vi "MotionMagicGoTo.vi"(7 "Reset":bool, 8 "error in (no error)":errorcluster, 9 "Offset(deg)":dbl, 10 "Distance(in)":dbl, 11 "Pod Drive in":refnum<class "Pod Drive.lvclass">) -> (0 "error out":errorcluster, 2 "Enum":T1=enum."ArcToTarget", 3 "Pod Drive out":refnum<class "Pod Drive.lvclass">)   [LabVIEW 2018, in "Drive.lvlib" / "Pod Drive.lvclass"]
uses:
  Pod Drive.lvclass
  Controls/AutoDeliverStateMachine.ctl
  <vilib>/Rock Robotics/WPI/ThirdParty/Phoenix-LabVIEW/Motor Controller/Controls/CTRE_Phoenix_MotorControl_ControlMode.ctl
  Pod Drive.lvclass/Pod Drive.ctl
  <vilib>/Rock Robotics/WPI/ThirdParty/Phoenix-LabVIEW/Motor Controller/Get/CTRE_Phoenix_MotorController_GetSelectedSensorData.vi
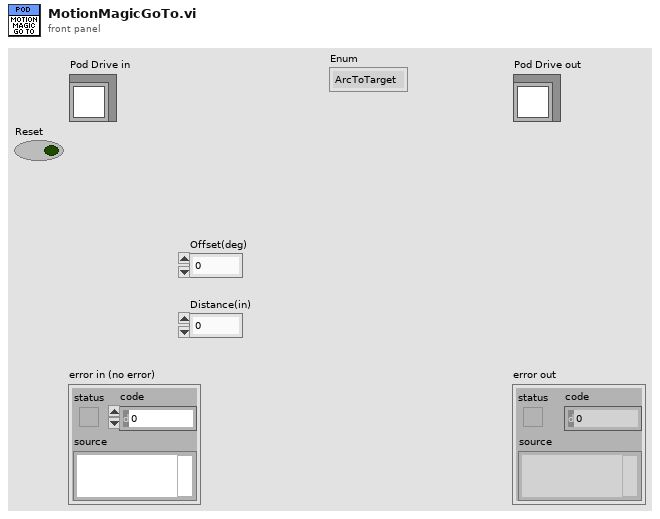
[diagram p1: front panel]
types:
  T1 = typedef "AutoDeliverStateMachine.ctl" = enum16{"Finish", "ArcToTarget", "TurnToTarget"}
  T2 = enum16{"DemandType_Neutral", "DemandType_AuxPID", "DemandType_ArbitraryFeedForward"}
  T3 = typedef "CTRE_Phoenix_MotorControl_ControlMode.ctl" = u16
  T4 = typedef "WPI_MotorControlDeviceRef.ctl" = cluster{"DeviceStatus":errorcluster, "Type":T5, "PWM":cluster{"PWM Channel":T6, "DeadBand":T7}, "CAN":cluster{"Device Number":u8, "SetOutput VI Ref":variant, "GetOutput VI Ref":variant, "Enable VI Ref":variant, "Disable VI Ref":variant, "Data":variant}, "Invert":bool, "DIO PWM":cluster{"PWM \"Enable\" Channel":T6, "DIOChannel":T8, "PWM Rate":dbl}}
  T5 = typedef "WPI_MotorControlType.ctl" = enum16{"PWM", "CAN", "DIO PWM"}
  T6 = typedef "FPGA_DIOPWMChannel.ctl" = enum8{"PWM 0", "PWM 1", "PWM 2", "PWM 3", "PWM 4", "PWM 5", "PWM 6", "PWM 7", "PWM 8", "PWM 9", "PWM MXP 0", "PWM MXP 1", "PWM MXP 2", "PWM MXP 3", "PWM MXP 4", "PWM MXP 5", "PWM MXP 6", "PWM MXP 7", "PWM MXP 8", "PWM MXP 9", "Invalid"}
  T7 = typedef "WPI_PWMDeadband.ctl" = cluster{"Name":string, "maxPositivePwm":i32, "minPositivePwm":i32, "centerPwm":i32, "maxNegativePwm":i32, "minNegativePwm":i32, "angularRange":u16}
  T8 = typedef "FPGA_DIOChannel.ctl" = enum8{"DIO 0", "DIO 1", "DIO 2", "DIO 3", "DIO 4", "DIO 5", "DIO 6", "DIO 7", "DIO 8", "DIO 9", "DIO MXP 0", "DIO MXP 1", "DIO MXP 2", "DIO MXP 3", "DIO MXP 4", "DIO MXP 5", "DIO MXP 6", "DIO MXP 7", "DIO MXP 8", "DIO MXP 9", "DIO MXP 10", "DIO MXP 11", "DIO MXP 12", "DIO MXP 13", "DIO MXP 14", "DIO MXP 15", "SPI Port CS1", "SPI Port CS2", "SPI Port CS3", "SPI Port MISO", "SPI Port MOSI", "Invalid"}
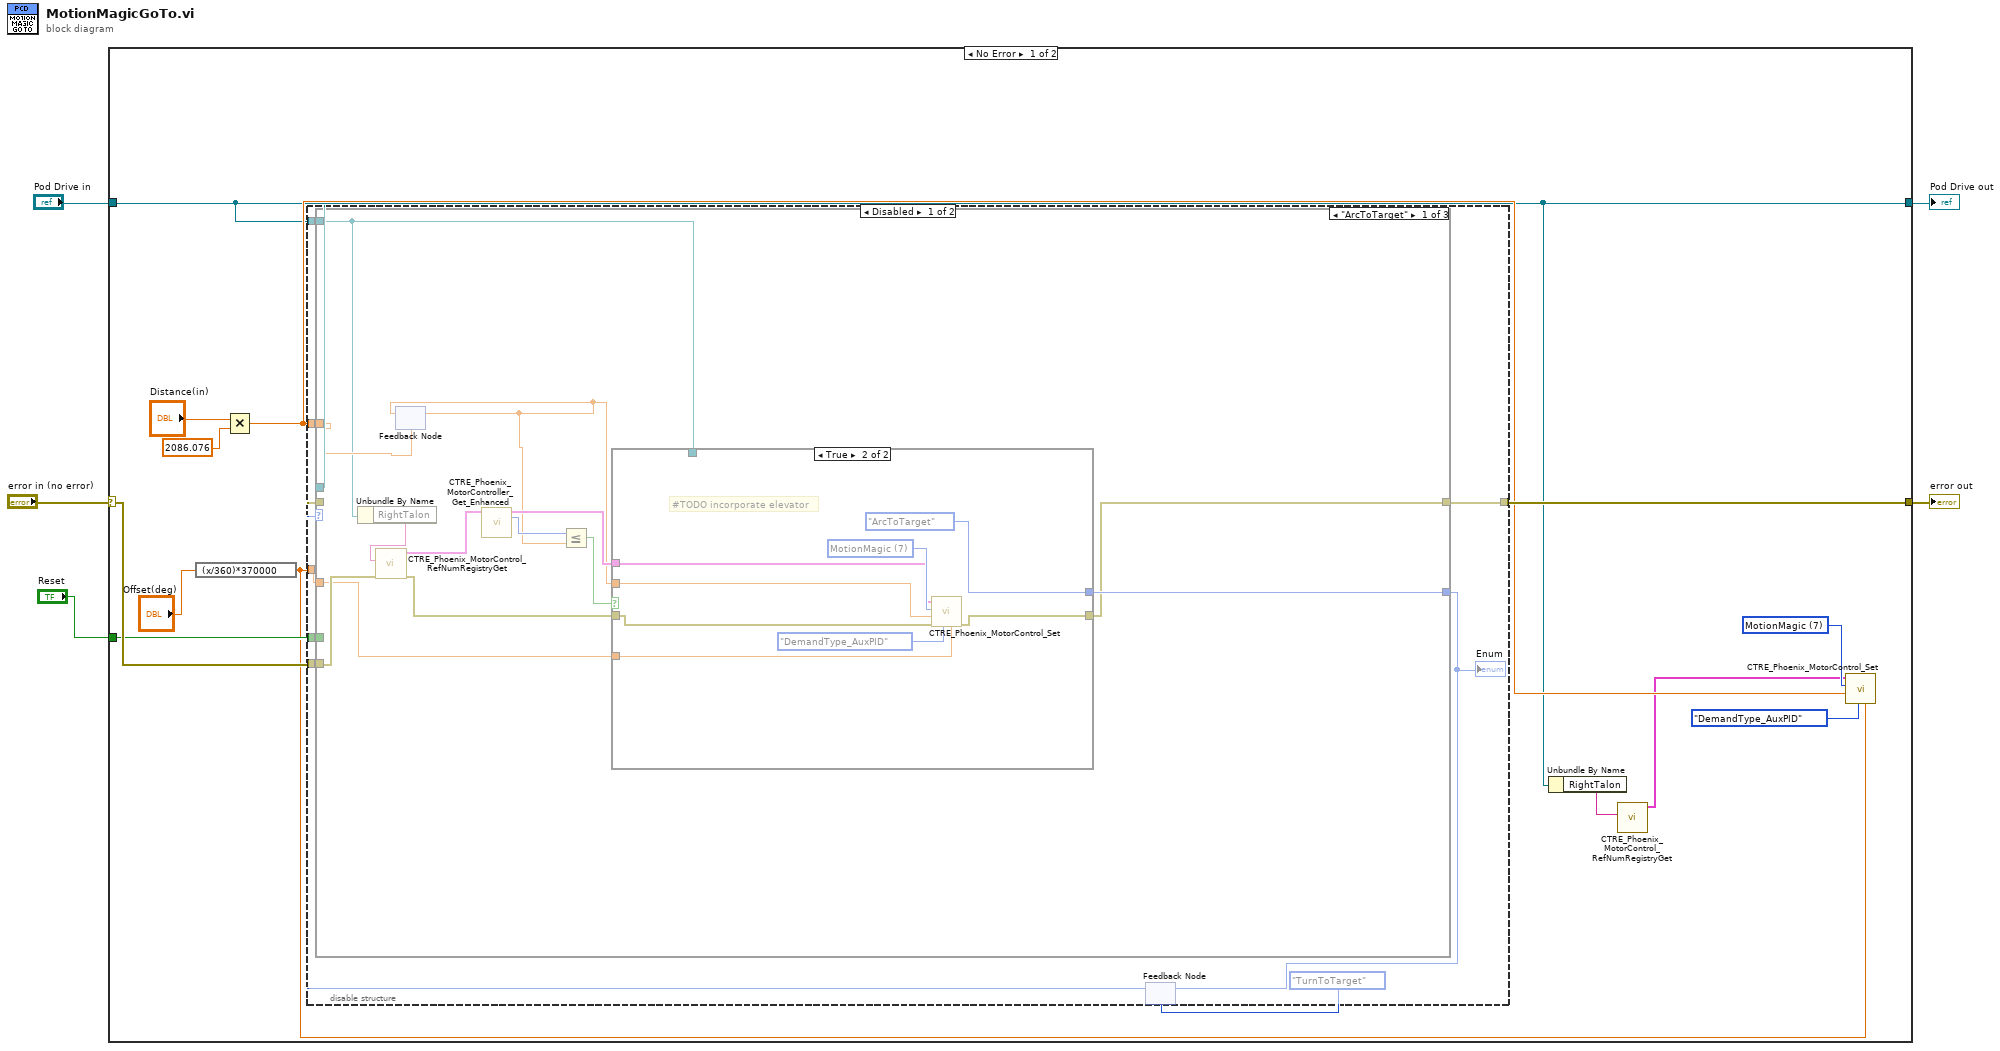
[diagram p0: block diagram]
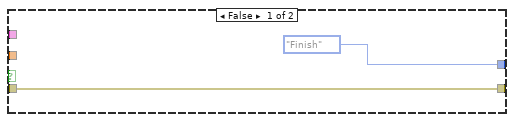
[diagram p2: hidden frame]
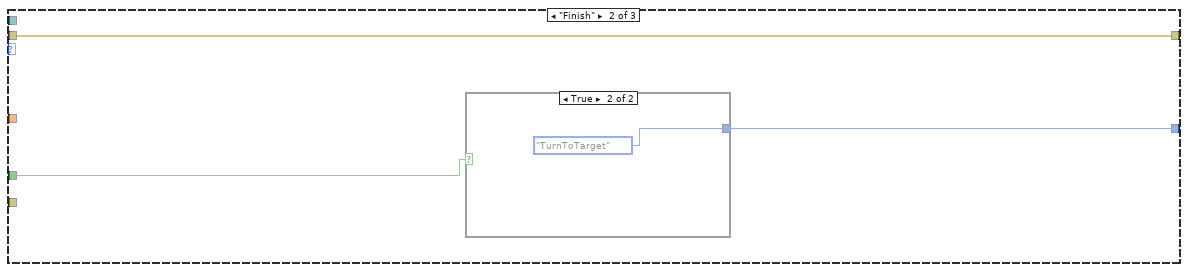
[diagram p3: hidden frame]
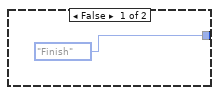
[diagram p4: hidden frame]
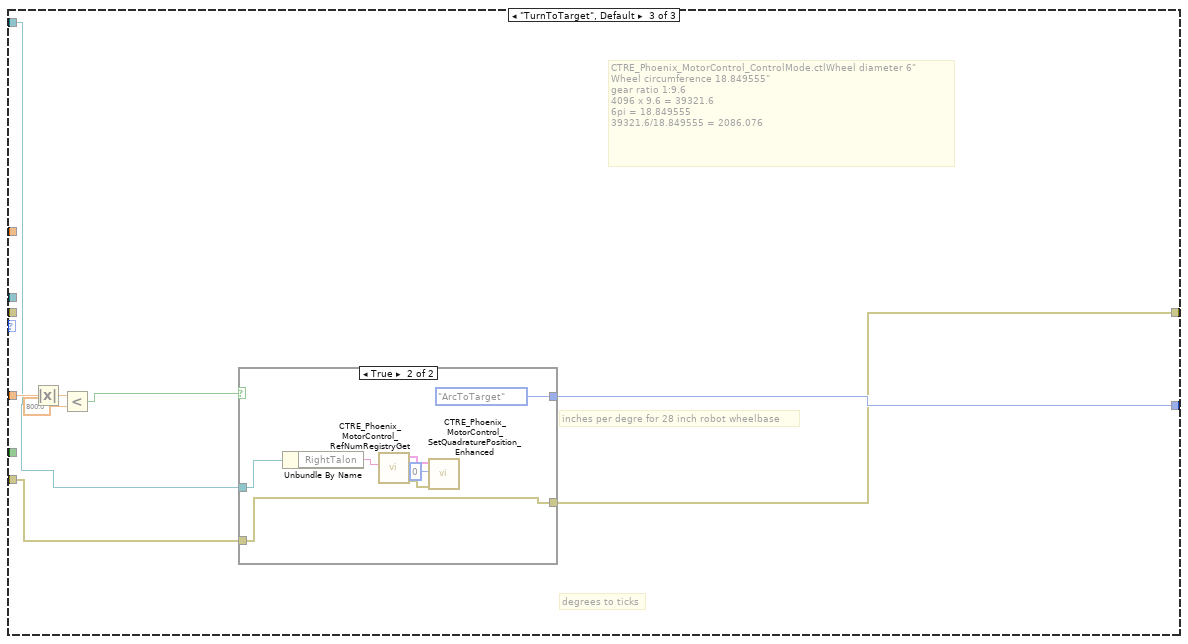
[diagram p5: hidden frame]
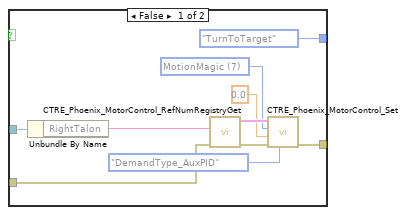
[diagram p6: hidden frame]
diagram:
  n1 = case shown="No Error" "error in (no error)" {
    selector: "error in (no error)" -> [w14 w82]
    tunnel: [w18 w82] -> w4
    tunnel: [w8 w81] -> w2
    tunnel: "Pod Drive in" -> [w8 w81]
    tunnel: "Reset" -> [w13 _]
    frame No Error {
      w11 = T3 7 items=["PercentOutput"=0, "Position"=1, "Velocity"=2, "Current"=3, "Follower"=5, "MotionProfile"=6, "MotionMagic"=7, "MotionProfileArc"=10, "Disabled"=15] ("Control Mode")
      n2 = expression code="(x/360)*370000"("Offset(deg)") -> (w9:dbl)
      n3 = Multiply(x="Distance(in)", y=2086.076) -> (x*y=w10:dbl)
      n4 = disable-structure shown="Disabled" {
        disable-tunnel: [w27 _] -> w18
        disable-tunnel: w10 -> [w24 _]
        disable-tunnel: w9 -> [w23 _]
        disable-tunnel: w14 -> [w22 _]
        disable-tunnel: w8 -> [w21 _]
        disable-tunnel: w13 -> [w19 _]
        frame Disabled {
          n5 = feedback #1(AutoDeliverStateMachine."TurnToTarget") -> (w25:T1)
          n6 = case shown="\"ArcToTarget\"" w25 {
            tunnel: w21 -> [_ _ _]
            tunnel: w22 -> [_ w53 _]
            tunnel: [w28 w53 w57] -> w27
            tunnel: w24 -> [w37 _ _]
            tunnel: w23 -> [w39 _ w63]
            tunnel: [w38 w51 w59] -> w20
            tunnel: w22 -> [w40 _ w58]
            tunnel: w21 -> [w36 _ w56]
            tunnel: w19 -> [_ w52 _]
            frame "ArcToTarget" {
              n7 = Unbundle By Name(w36) -> ("RightTalon"=w34:string)
              n8 = call <vilib>:"CTRE_Phoenix_MotorControl_RefNumRegistryGet.vi"("error in (no error)"=w40, "refnum name"=w34) -> ("error out"=w35:errorcluster, "PhoenixMotorControlDevRef"=w33:T4)  [unwired: 8 in]
              n9 = feedback #2(w37) -> (w29:dbl)
              n10 = feedback-in #2(w29) -> ()
              n11 = call-poly <vilib>:"CTRE_Phoenix_MotorController_Get_Enhanced.vi"("PhoenixMotorControlDevRef"=w33) -> ("PhoenixMotorControlDevRef"=w32:T4, "Position (Raw Sensor Units)"=w31:i32)  [unwired: 11 in, 2 out]
              n12 = Less Or Equal?(x=w31, y=w29) -> (x <= y?=w30:bool)
              n13 = case shown="True" w30 {
                tunnel: w29 -> [_ w48]
                tunnel: w39 -> [_ w47]
                tunnel: [AutoDeliverStateMachine."Finish" AutoDeliverStateMachine."ArcToTarget"] -> w38
                tunnel: w36 -> [_ _]
                tunnel: w35 -> [w41 w45]
                tunnel: w32 -> [_ w44]
                tunnel: [w41 w43] -> w28
                frame False {
                }
                frame True {
                  w49 = T3 7 items=["PercentOutput"=0, "Position"=1, "Velocity"=2, "Current"=3, "Follower"=5, "MotionProfile"=6, "MotionMagic"=7, "MotionProfileArc"=10, "Disabled"=15] ("Control Mode")
                  # "#TODO incorporate elevator"
                  n14 = call <vilib>:"CTRE_Phoenix_MotorControl_Set.vi"("Demand1"=w47, "DemandType"=T2."DemandType_AuxPID", "error in (no error)"=w45, "Output"=w48, "Control Mode"=w49, "PhoenixMotorControlDevRef"=w44) -> ("error out"=w43:errorcluster)  [unwired: 4 in, 1 out]
                }
              }
            }
            frame "Finish" {
              n15 = case shown="True" w52 {
                tunnel: [AutoDeliverStateMachine."Finish" AutoDeliverStateMachine."TurnToTarget"] -> w51
                frame False {
                }
                frame True {
                }
              }
            }
            frame "TurnToTarget", Default {
              # "inches per degre for 28 inch robot wheelbase"
              # "CTRE_Phoenix_MotorControl_ControlMode.ctlWheel diameter 6\"\nWheel circumference 18.849555\"\ngear ratio 1:9.6\n4096 x 9.6 = 39321.6\n6pi = 18.849555\n39321.6/18.849555 = 2086.076"
              # "degrees to ticks"
              n16 = Absolute Value(x=w63) -> (abs(x)=w61:dbl)
              n17 = Less?(x=w61, y=800.0) -> (x < y?=w60:bool)
              n18 = case shown="True" w60 {
                tunnel: [AutoDeliverStateMachine."TurnToTarget" AutoDeliverStateMachine."ArcToTarget"] -> w59
                tunnel: w58 -> [w70 w79]
                tunnel: [w67 w79] -> w57
                tunnel: w56 -> [w66 w78]
                frame False {
                  w64 = T3 7 items=["PercentOutput"=0, "Position"=1, "Velocity"=2, "Current"=3, "Follower"=5, "MotionProfile"=6, "MotionMagic"=7, "MotionProfileArc"=10, "Disabled"=15] ("Control Mode")
                  n19 = Unbundle By Name(w66) -> ("RightTalon"=w65:string)
                  n20 = call <vilib>:"CTRE_Phoenix_MotorControl_RefNumRegistryGet.vi"("error in (no error)"=w70, "refnum name"=w65) -> ("error out"=w71:errorcluster, "PhoenixMotorControlDevRef"=w72:T4)  [unwired: 8 in]
                  n21 = call <vilib>:"CTRE_Phoenix_MotorControl_Set.vi"("DemandType"=T2."DemandType_AuxPID", "error in (no error)"=w71, "Output"=0.0, "Control Mode"=w64, "PhoenixMotorControlDevRef"=w72) -> ("error out"=w67:errorcluster)  [unwired: 5 in, 1 out]
                }
                frame True {
                  n22 = Unbundle By Name(w78) -> ("RightTalon"=w77:string)
                  n23 = call <vilib>:"CTRE_Phoenix_MotorControl_RefNumRegistryGet.vi"("refnum name"=w77) -> ("error out"=w76:errorcluster, "PhoenixMotorControlDevRef"=w75:T4)  [unwired: 9 in]
                  n24 = call <vilib>:"CTRE_Phoenix_MotorControl_SetQuadraturePosition_Enhanced.vi"("error in (no error)"=w76, "New Position"=0, "PhoenixMotorControlDevRef"=w75) -> ()  [unwired: 7 in, 2 out]
                }
              }
            }
          }
          "Enum" <- w20
          n25 = feedback-in #1(w20) -> ()
        }
        frame Enabled {
        }
      }
      n26 = Unbundle By Name(w8) -> ("RightTalon"=w7:string)
      n27 = call <vilib>:"CTRE_Phoenix_MotorControl_RefNumRegistryGet.vi"("refnum name"=w7) -> ("PhoenixMotorControlDevRef"=w6:T4)  [unwired: 9 in, 1 out]
      n28 = call <vilib>:"CTRE_Phoenix_MotorControl_Set.vi"("Demand1"=w9, "DemandType"=T2."DemandType_AuxPID", "Output"=w10, "Control Mode"=w11, "PhoenixMotorControlDevRef"=w6) -> ()  [unwired: 5 in, 2 out]
    }
    frame Error {
    }
  }
  "error out" <- w4
  "Pod Drive out" <- w2
